vi "Supervisor.vi"() -> ()   [LabVIEW 2017]
panel:
  in  "MATLAB Active":bool
  in  "Stop Supervisor":bool
  in  "Action Recorder ON":bool
  # "Supervisor"
  # "Management Box"
  # "Procedures"
  # "Shared Information"
  # "Information and Action Requests"
  # "NOAH - Networked Operator Analytical Helper"
  # "Fault Information"
  # "Analytics"
  # "Pinned Items"
  # "Grey-Box"
  # "Data-Driven"
  # "Analytical"
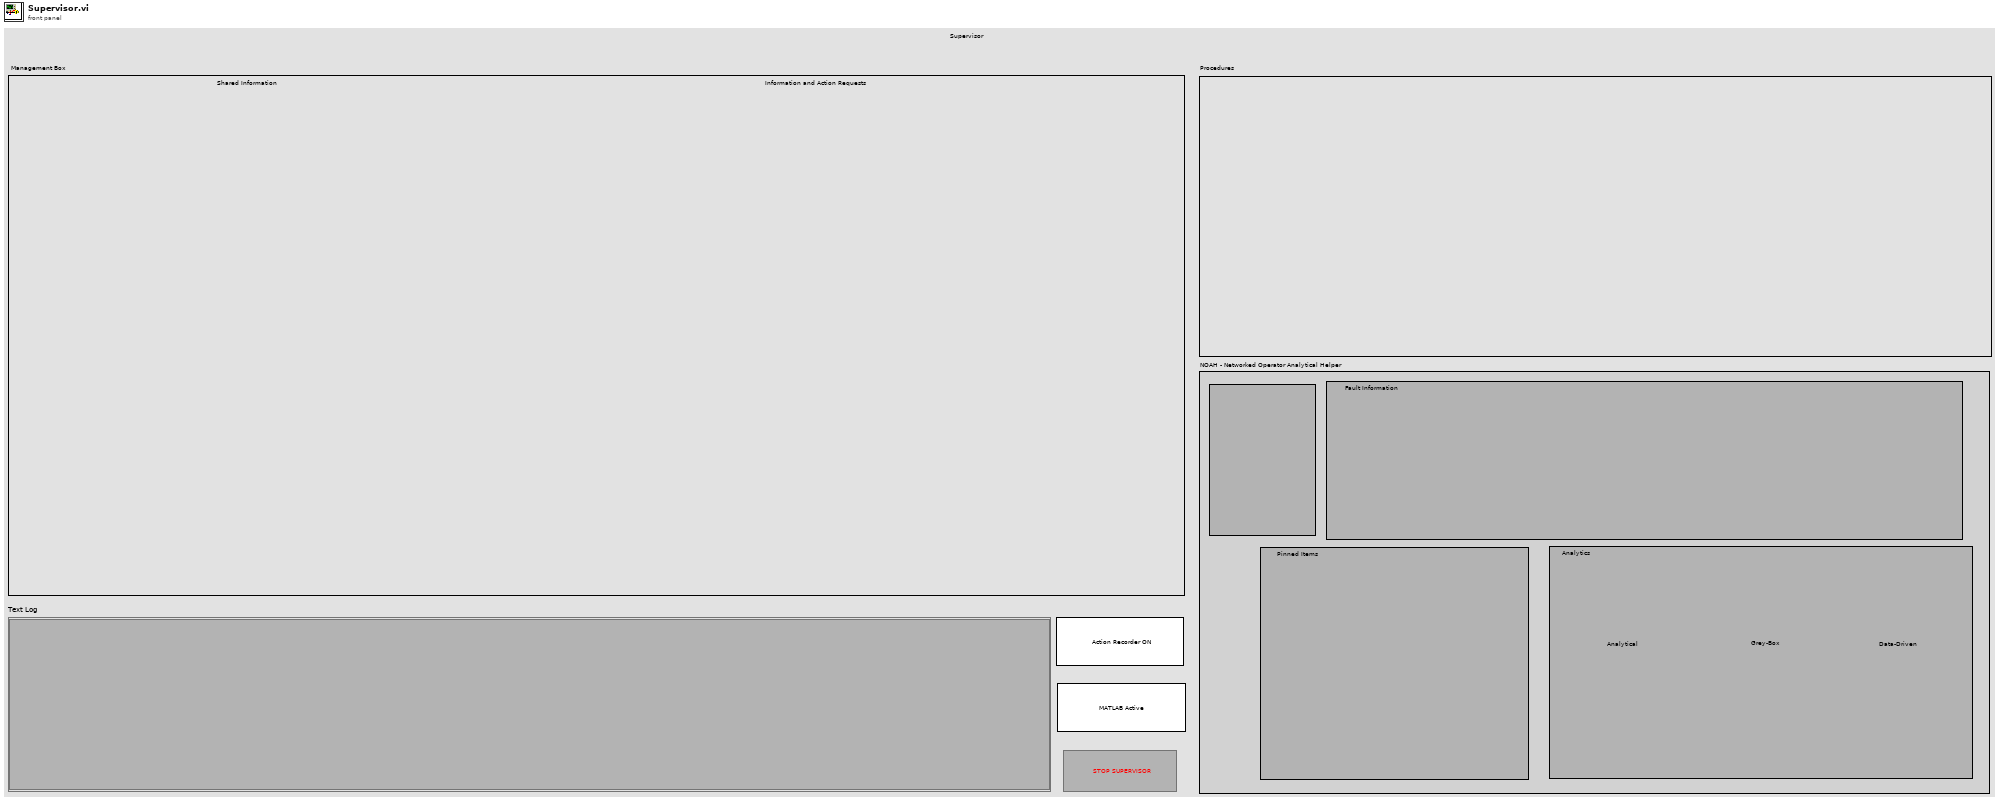
[diagram p1: front panel]
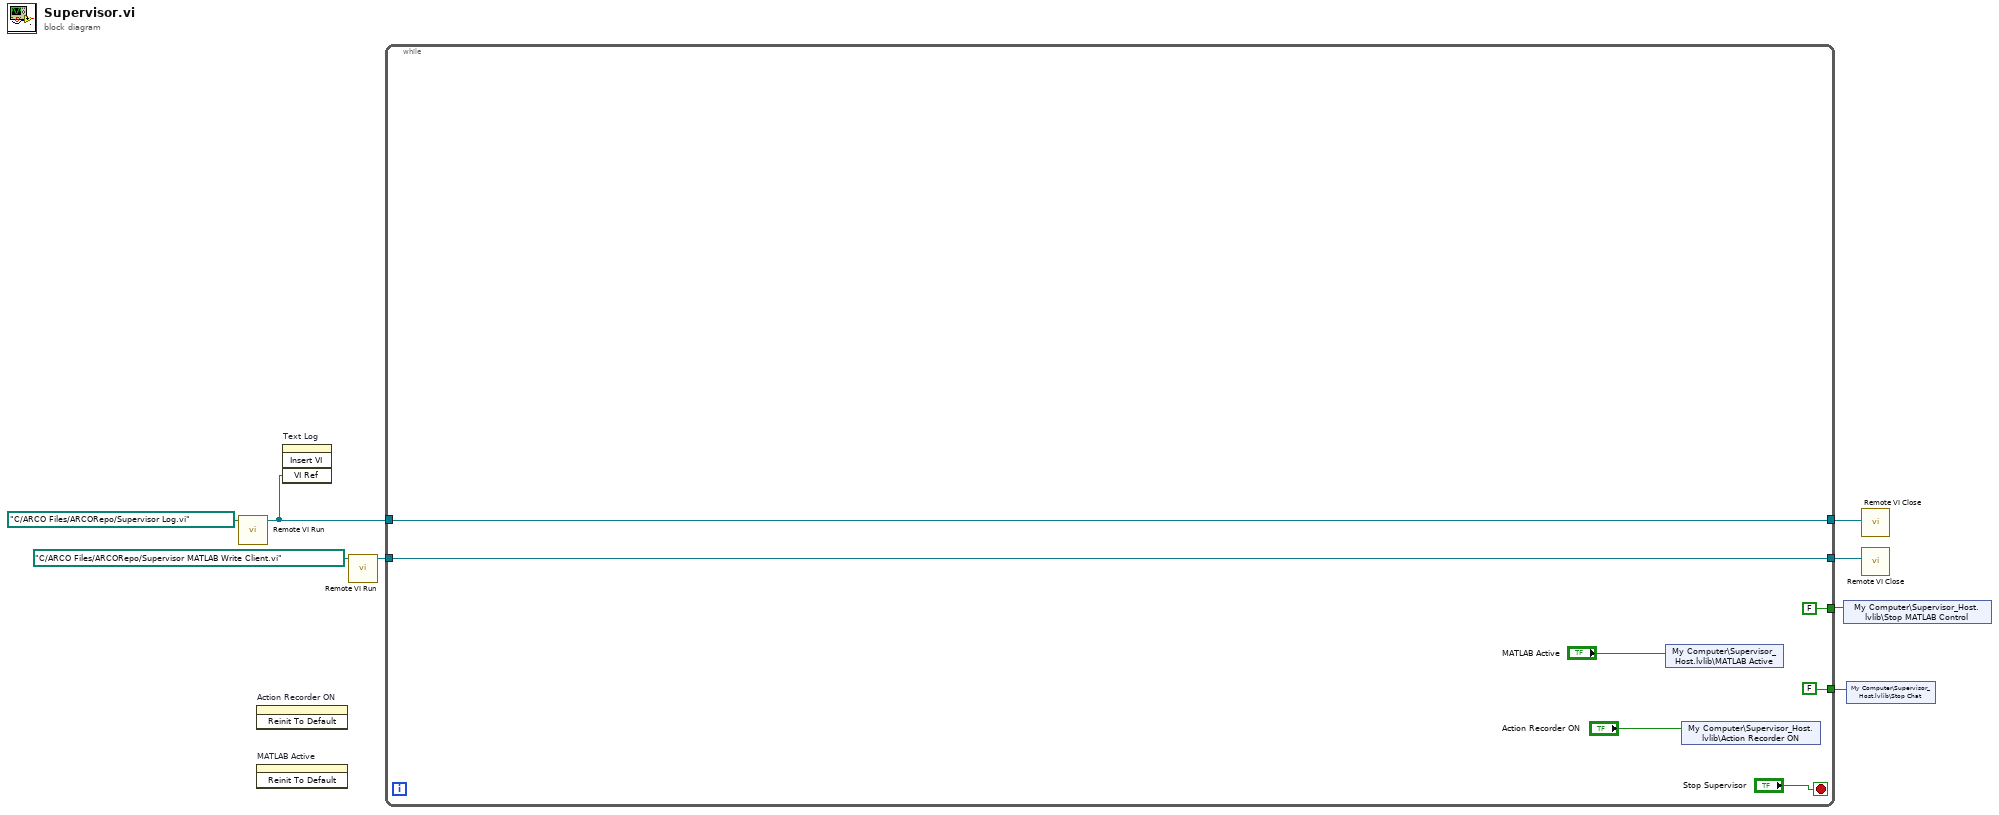
[diagram p0: block diagram]
diagram:
  n1 = call "Remote VI Run.vi"("VI Path"=path "C:/ARCO Files/ARCORepo/Supervisor Log.vi") -> ("VI Reference"=w7:refnum<vi>)  [unwired: 10 in]
  n2 = invoke on="Action Recorder ON" class="Bool (strict)" method="Reinit To Default"() -> ()  [unwired: 3 in, 3 out]
  n3 = invoke on="MATLAB Active" class="Bool (strict)" method="Reinit To Default"() -> ()  [unwired: 3 in, 3 out]
  n4 = invoke on="Text Log" class="SubPnl" method="Insert VI"("VI Ref"=w7) -> ()  [unwired: 3 in, 4 out]
  n5 = call "Remote VI Run.vi"("VI Path"=path "C:/ARCO Files/ARCORepo/Supervisor MATLAB Write Client.vi") -> ("VI Reference"=w4:refnum<vi>)  [unwired: 10 in]
  n6 = while {
    tunnel: w7 -> [w14]
    tunnel: [w14] -> w6
    tunnel: w4 -> [w11]
    tunnel: [w11] -> w3
    tunnel: [FALSE] -> w2
    tunnel: [FALSE] -> w1
    stop <- "Stop Supervisor" stop-if-true
    n7 = shared-variable "My Computer\\Supervisor_Host.lvlib\\MATLAB Active"("MATLAB Active") -> ()  [unwired: 1 in, 1 out]
    n8 = shared-variable "My Computer\\Supervisor_Host.lvlib\\Action Recorder ON"("Action Recorder ON") -> ()  [unwired: 1 in, 1 out]
  }
  n9 = shared-variable "My Computer\\Supervisor_Host.lvlib\\Stop MATLAB Control"(w1) -> ()  [unwired: 1 in, 1 out]
  n10 = shared-variable "My Computer\\Supervisor_Host.lvlib\\Stop Chat"(w2) -> ()  [unwired: 1 in, 1 out]
  n11 = call "Remote VI Close.vi"("reference"=w6) -> ()  [unwired: 10 in, 1 out]
  n12 = call "Remote VI Close.vi"("reference"=w3) -> ()  [unwired: 10 in, 1 out]
